vi "MicrofluidicChipControl.vi"() -> ()   [LabVIEW 2023]
uses:
  <vilib>/LabVIEW Interface for Arduino/Type Defs/Board Type.ctl
  <vilib>/LabVIEW Interface for Arduino/Type Defs/Pin Mode.ctl
  <vilib>/LabVIEW Interface for Arduino/LabVIEW Interface for Arduino.lvlib
panel:
  in  "Wait(ms)":dbl=200.0
  in  "Port":refnum<visa-resource-name>="COM3"
  in  "?":string=" BSV4_b"
  in  "?":string=" BSV3_b"
  in  "?":string=" BSV2_b"
  in  "?":string="BSV1_b"
  in  "?":string=" "
  in  "?":string=" "
  in  "?":string="BCV_r"
  in  "?":string="APV_r"
  in  "?":string="CCV"
  in  "?":string="MV"
  in  "?":string="NV"
  in  "?":string="BCV"
  in  "?":string="BV"
  in  "?":string="CRV"
  in  "?":string="SV"
  in  "?":string="SPV"
  in  "?":string="BSV8"
  in  "?":string="BSV7"
  in  "?":string="BSV6"
  in  "?":string="BSV5"
  in  "?":string="BSV4"
  in  "?":string="BSV3"
  in  "?":string="BSV2"
  in  "?":string="BSV1"
  in  "?":string=" COV"
  in  "?":string=" "
  in  "?":string="CCV"
  in  "?":string="CSV4"
  in  "?":string="CSV3"
  in  "?":string="CSV2"
  in  "?":string="CSV1"
  in  "?":string="APV_l"
  in  "D8":bool
  in  "D7":bool
  in  "D6":bool
  in  "D5":bool
  in  "D4":bool
  in  "D3":bool
  in  "D2":bool
  in  "D1":bool
  in  "C8":bool
  in  "C7":bool
  in  "C6":bool
  in  "C5":bool
  in  "C4":bool
  in  "C3":bool
  in  "C2":bool
  in  "C1":bool
  in  "B8":bool
  in  "B7":bool
  in  "B6":bool
  in  "B5":bool
  in  "B4":bool
  in  "B3":bool
  in  "B2":bool
  in  "B1":bool
  in  "A8":bool
  in  "A7":bool
  in  "A6":bool
  in  "A5":bool
  in  "A4":bool
  in  "A3":bool
  in  "A2":bool
  in  "A1":bool
  in  "stop":bool
  in  "Start Mixing":bool
  # "Laboratory of Microtechnologies Applied to Biomedicine"
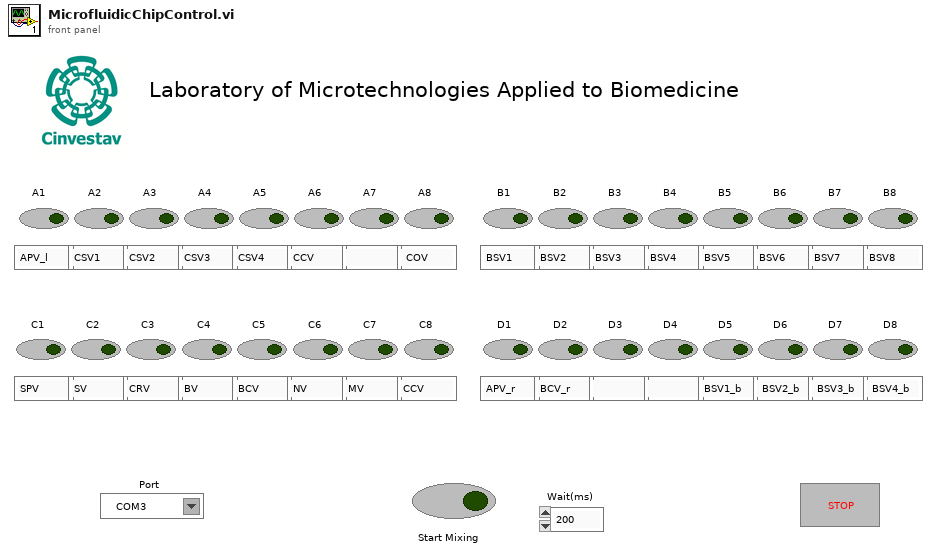
[diagram p1: front panel]
types:
  T1 = typedef "LabVIEW Interface for Arduino.lvlib/Board Type.ctl" = enum16{"Uno", "Dimuelanove w/Atmega 328", "Mega 2560"}
  T2 = typedef "LabVIEW Interface for Arduino.lvlib/Arduino Resource.ctl" = cluster{"VISA resource":refnum<visa-resource-name>, "Board Type":T1, "Connection Type":enum8{"USB / Serial"}, "Bytes Per Packet (15)":u8}
  T3 = typedef "LabVIEW Interface for Arduino.lvlib/Pin Mode.ctl" = enum8{"Input", "Output"}
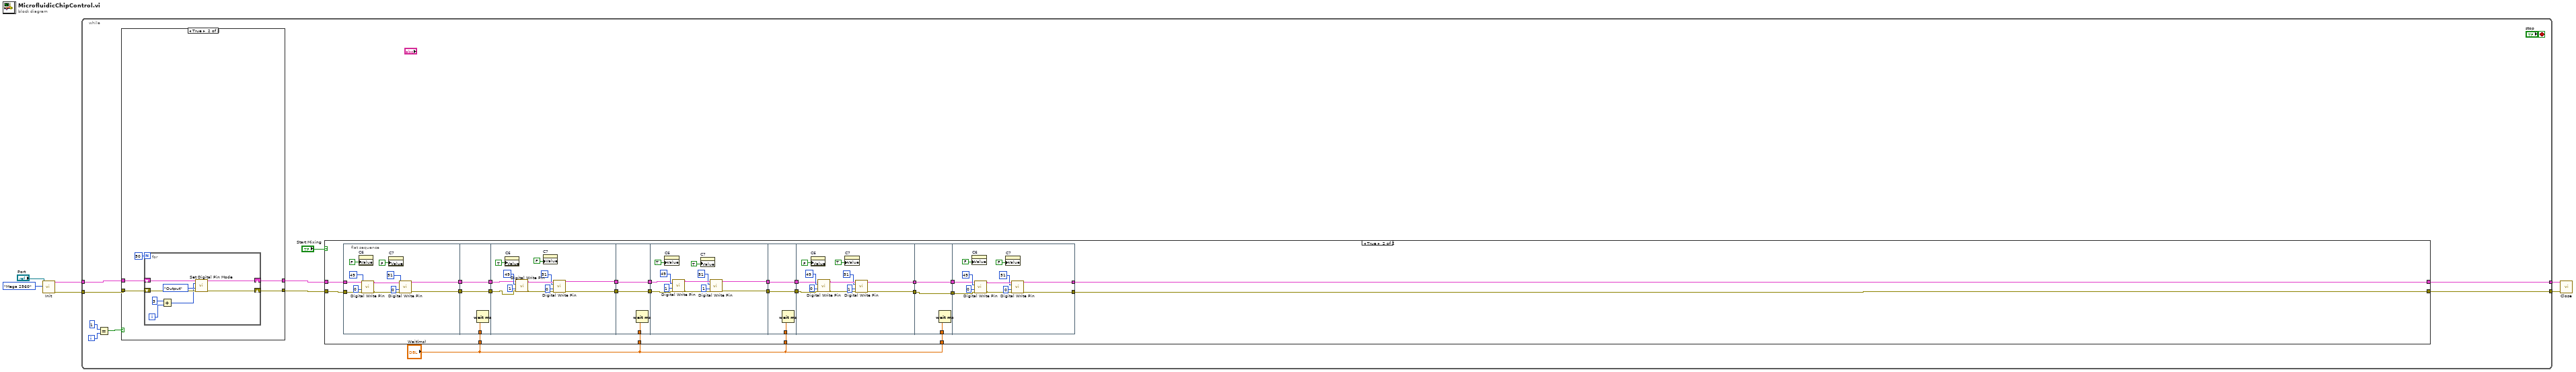
[diagram p0: block diagram]
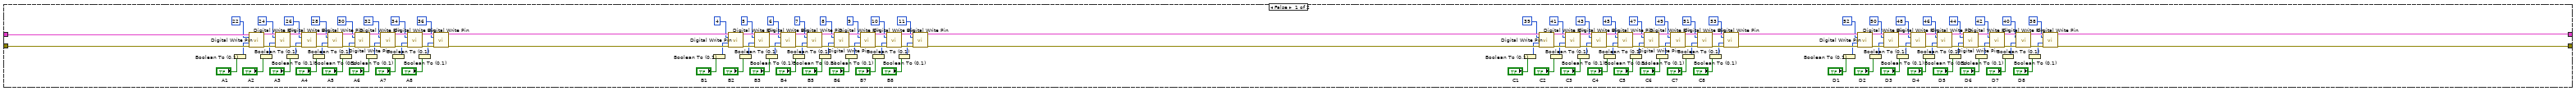
[diagram p2: hidden frame]
diagram:
  n1 = call <vilib>:"Init.vi"("VISA resource"="Port", "Board Type (Uno)"=Board_Type."Mega 2560") -> ("Arduino Resource"=w4:T2, "error out"=w3:errorcluster)  [unwired: 16 in]
  n2 = while {
    tunnel: w4 -> [w15]
    tunnel: w3 -> [w11]
    tunnel: [w10] -> w1
    tunnel: [w9] -> w2
    i -> [w18]
    stop <- "stop" stop-if-true
    n3 = Equal?(x=1, y=w18) -> (x = y?=w16:bool)
    n4 = case shown="True" w16 {
      tunnel: w15 -> [w278 w282]
      tunnel: w11 -> [w277 w281]
      tunnel: [w278 w280] -> w13
      tunnel: [w277 w279] -> w12
      frame False {
      }
      frame True {
        n5 = for {
          N: 50 -> [_]
          shift-right: [w287] -> w280
          shift-left: w282 -> [w290]
          shift-right: [w288] -> w279
          shift-left: w281 -> [w289]
          i -> [w286]
          n6 = Add(x=3, y=w286) -> (x+y=w285:i32)
          n7 = call <vilib>:"Set Digital Pin Mode.vi"("Arduino Resource"=w290, "Digital I/O Pin"=w285, "Pin Mode (Input)"=Pin_Mode."Output", "error in"=w289) -> ("Arduino Resource"=w287:T2, "error out"=w288:errorcluster)  [unwired: 10 in]
        }
      }
    }
    n8 = case shown="True" "Start Mixing" {
      tunnel: w13 -> [w180 w194]
      tunnel: w12 -> [w179 w193]
      tunnel: [w20 w192] -> w9
      tunnel: [w19 w191] -> w10
      tunnel: "Wait(ms)" -> [_ w190]
      tunnel: "Wait(ms)" -> [_ w189]
      tunnel: "Wait(ms)" -> [_ w188]
      tunnel: "Wait(ms)" -> [_ w181]
      frame False {
        n9 = Boolean To (0,1)(Boolean="A1") -> (0, 1=w116:i16)
        n10 = call <vilib>:"Digital Write Pin.vi"("Arduino Resource"=w180, "Digital I/O Pin (0)"=u8 22, "Value (0)"=w116, "error in"=w179) -> ("Arduino Resource"=w178:T2, "error out"=w177:errorcluster)  [unwired: 10 in]
        n11 = Boolean To (0,1)(Boolean="A2") -> (0, 1=w115:i16)
        n12 = call <vilib>:"Digital Write Pin.vi"("Arduino Resource"=w178, "Digital I/O Pin (0)"=u8 24, "Value (0)"=w115, "error in"=w177) -> ("Arduino Resource"=w176:T2, "error out"=w175:errorcluster)  [unwired: 10 in]
        n13 = Boolean To (0,1)(Boolean="A3") -> (0, 1=w114:i16)
        n14 = call <vilib>:"Digital Write Pin.vi"("Arduino Resource"=w176, "Digital I/O Pin (0)"=u8 26, "Value (0)"=w114, "error in"=w175) -> ("Arduino Resource"=w174:T2, "error out"=w173:errorcluster)  [unwired: 10 in]
        n15 = Boolean To (0,1)(Boolean="A4") -> (0, 1=w113:i16)
        n16 = call <vilib>:"Digital Write Pin.vi"("Arduino Resource"=w174, "Digital I/O Pin (0)"=u8 28, "Value (0)"=w113, "error in"=w173) -> ("Arduino Resource"=w172:T2, "error out"=w171:errorcluster)  [unwired: 10 in]
        n17 = Boolean To (0,1)(Boolean="A5") -> (0, 1=w112:i16)
        n18 = call <vilib>:"Digital Write Pin.vi"("Arduino Resource"=w172, "Digital I/O Pin (0)"=u8 30, "Value (0)"=w112, "error in"=w171) -> ("Arduino Resource"=w170:T2, "error out"=w169:errorcluster)  [unwired: 10 in]
        n19 = Boolean To (0,1)(Boolean="A6") -> (0, 1=w111:i16)
        n20 = call <vilib>:"Digital Write Pin.vi"("Arduino Resource"=w170, "Digital I/O Pin (0)"=u8 32, "Value (0)"=w111, "error in"=w169) -> ("Arduino Resource"=w168:T2, "error out"=w167:errorcluster)  [unwired: 10 in]
        n21 = Boolean To (0,1)(Boolean="A7") -> (0, 1=w110:i16)
        n22 = call <vilib>:"Digital Write Pin.vi"("Arduino Resource"=w168, "Digital I/O Pin (0)"=u8 34, "Value (0)"=w110, "error in"=w167) -> ("Arduino Resource"=w166:T2, "error out"=w165:errorcluster)  [unwired: 10 in]
        n23 = Boolean To (0,1)(Boolean="A8") -> (0, 1=w109:i16)
        n24 = call <vilib>:"Digital Write Pin.vi"("Arduino Resource"=w166, "Digital I/O Pin (0)"=u8 36, "Value (0)"=w109, "error in"=w165) -> ("Arduino Resource"=w164:T2, "error out"=w163:errorcluster)  [unwired: 10 in]
        n25 = Boolean To (0,1)(Boolean="B1") -> (0, 1=w108:i16)
        n26 = call <vilib>:"Digital Write Pin.vi"("Arduino Resource"=w164, "Digital I/O Pin (0)"=u8 4, "Value (0)"=w108, "error in"=w163) -> ("Arduino Resource"=w162:T2, "error out"=w161:errorcluster)  [unwired: 10 in]
        n27 = Boolean To (0,1)(Boolean="B2") -> (0, 1=w107:i16)
        n28 = call <vilib>:"Digital Write Pin.vi"("Arduino Resource"=w162, "Digital I/O Pin (0)"=u8 5, "Value (0)"=w107, "error in"=w161) -> ("Arduino Resource"=w160:T2, "error out"=w159:errorcluster)  [unwired: 10 in]
        n29 = Boolean To (0,1)(Boolean="B3") -> (0, 1=w106:i16)
        n30 = call <vilib>:"Digital Write Pin.vi"("Arduino Resource"=w160, "Digital I/O Pin (0)"=u8 6, "Value (0)"=w106, "error in"=w159) -> ("Arduino Resource"=w157:T2, "error out"=w158:errorcluster)  [unwired: 10 in]
        n31 = Boolean To (0,1)(Boolean="B4") -> (0, 1=w105:i16)
        n32 = call <vilib>:"Digital Write Pin.vi"("Arduino Resource"=w157, "Digital I/O Pin (0)"=u8 7, "Value (0)"=w105, "error in"=w158) -> ("Arduino Resource"=w156:T2, "error out"=w155:errorcluster)  [unwired: 10 in]
        n33 = Boolean To (0,1)(Boolean="B5") -> (0, 1=w104:i16)
        n34 = call <vilib>:"Digital Write Pin.vi"("Arduino Resource"=w156, "Digital I/O Pin (0)"=u8 8, "Value (0)"=w104, "error in"=w155) -> ("Arduino Resource"=w154:T2, "error out"=w153:errorcluster)  [unwired: 10 in]
        n35 = Boolean To (0,1)(Boolean="B6") -> (0, 1=w103:i16)
        n36 = call <vilib>:"Digital Write Pin.vi"("Arduino Resource"=w154, "Digital I/O Pin (0)"=u8 9, "Value (0)"=w103, "error in"=w153) -> ("Arduino Resource"=w152:T2, "error out"=w151:errorcluster)  [unwired: 10 in]
        n37 = Boolean To (0,1)(Boolean="B7") -> (0, 1=w102:i16)
        n38 = call <vilib>:"Digital Write Pin.vi"("Arduino Resource"=w152, "Digital I/O Pin (0)"=u8 10, "Value (0)"=w102, "error in"=w151) -> ("Arduino Resource"=w150:T2, "error out"=w149:errorcluster)  [unwired: 10 in]
        n39 = Boolean To (0,1)(Boolean="B8") -> (0, 1=w101:i16)
        n40 = call <vilib>:"Digital Write Pin.vi"("Arduino Resource"=w150, "Digital I/O Pin (0)"=u8 11, "Value (0)"=w101, "error in"=w149) -> ("Arduino Resource"=w118:T2, "error out"=w117:errorcluster)  [unwired: 10 in]
        n41 = Boolean To (0,1)(Boolean="C1") -> (0, 1=w100:i16)
        n42 = call <vilib>:"Digital Write Pin.vi"("Arduino Resource"=w118, "Digital I/O Pin (0)"=u8 39, "Value (0)"=w100, "error in"=w117) -> ("Arduino Resource"=w148:T2, "error out"=w147:errorcluster)  [unwired: 10 in]
        n43 = Boolean To (0,1)(Boolean="C2") -> (0, 1=w99:i16)
        n44 = call <vilib>:"Digital Write Pin.vi"("Arduino Resource"=w148, "Digital I/O Pin (0)"=u8 41, "Value (0)"=w99, "error in"=w147) -> ("Arduino Resource"=w146:T2, "error out"=w145:errorcluster)  [unwired: 10 in]
        n45 = Boolean To (0,1)(Boolean="C3") -> (0, 1=w98:i16)
        n46 = call <vilib>:"Digital Write Pin.vi"("Arduino Resource"=w146, "Digital I/O Pin (0)"=u8 43, "Value (0)"=w98, "error in"=w145) -> ("Arduino Resource"=w144:T2, "error out"=w143:errorcluster)  [unwired: 10 in]
        n47 = Boolean To (0,1)(Boolean="C4") -> (0, 1=w97:i16)
        n48 = call <vilib>:"Digital Write Pin.vi"("Arduino Resource"=w144, "Digital I/O Pin (0)"=u8 45, "Value (0)"=w97, "error in"=w143) -> ("Arduino Resource"=w142:T2, "error out"=w141:errorcluster)  [unwired: 10 in]
        n49 = Boolean To (0,1)(Boolean="C5") -> (0, 1=w96:i16)
        n50 = call <vilib>:"Digital Write Pin.vi"("Arduino Resource"=w142, "Digital I/O Pin (0)"=u8 47, "Value (0)"=w96, "error in"=w141) -> ("Arduino Resource"=w140:T2, "error out"=w139:errorcluster)  [unwired: 10 in]
        n51 = Boolean To (0,1)(Boolean="C6") -> (0, 1=w95:i16)
        n52 = call <vilib>:"Digital Write Pin.vi"("Arduino Resource"=w140, "Digital I/O Pin (0)"=u8 49, "Value (0)"=w95, "error in"=w139) -> ("Arduino Resource"=w138:T2, "error out"=w137:errorcluster)  [unwired: 10 in]
        n53 = Boolean To (0,1)(Boolean="C7") -> (0, 1=w94:i16)
        n54 = call <vilib>:"Digital Write Pin.vi"("Arduino Resource"=w138, "Digital I/O Pin (0)"=u8 51, "Value (0)"=w94, "error in"=w137) -> ("Arduino Resource"=w136:T2, "error out"=w135:errorcluster)  [unwired: 10 in]
        n55 = Boolean To (0,1)(Boolean="C8") -> (0, 1=w93:i16)
        n56 = call <vilib>:"Digital Write Pin.vi"("Arduino Resource"=w136, "Digital I/O Pin (0)"=u8 53, "Value (0)"=w93, "error in"=w135) -> ("Arduino Resource"=w134:T2, "error out"=w133:errorcluster)  [unwired: 10 in]
        n57 = Boolean To (0,1)(Boolean="D1") -> (0, 1=w92:i16)
        n58 = call <vilib>:"Digital Write Pin.vi"("Arduino Resource"=w134, "Digital I/O Pin (0)"=u8 52, "Value (0)"=w92, "error in"=w133) -> ("Arduino Resource"=w132:T2, "error out"=w131:errorcluster)  [unwired: 10 in]
        n59 = Boolean To (0,1)(Boolean="D2") -> (0, 1=w91:i16)
        n60 = call <vilib>:"Digital Write Pin.vi"("Arduino Resource"=w132, "Digital I/O Pin (0)"=u8 50, "Value (0)"=w91, "error in"=w131) -> ("Arduino Resource"=w130:T2, "error out"=w129:errorcluster)  [unwired: 10 in]
        n61 = Boolean To (0,1)(Boolean="D3") -> (0, 1=w90:i16)
        n62 = call <vilib>:"Digital Write Pin.vi"("Arduino Resource"=w130, "Digital I/O Pin (0)"=u8 48, "Value (0)"=w90, "error in"=w129) -> ("Arduino Resource"=w127:T2, "error out"=w128:errorcluster)  [unwired: 10 in]
        n63 = Boolean To (0,1)(Boolean="D4") -> (0, 1=w89:i16)
        n64 = call <vilib>:"Digital Write Pin.vi"("Arduino Resource"=w127, "Digital I/O Pin (0)"=u8 46, "Value (0)"=w89, "error in"=w128) -> ("Arduino Resource"=w126:T2, "error out"=w125:errorcluster)  [unwired: 10 in]
        n65 = Boolean To (0,1)(Boolean="D5") -> (0, 1=w88:i16)
        n66 = call <vilib>:"Digital Write Pin.vi"("Arduino Resource"=w126, "Digital I/O Pin (0)"=u8 44, "Value (0)"=w88, "error in"=w125) -> ("Arduino Resource"=w124:T2, "error out"=w123:errorcluster)  [unwired: 10 in]
        n67 = Boolean To (0,1)(Boolean="D6") -> (0, 1=w87:i16)
        n68 = call <vilib>:"Digital Write Pin.vi"("Arduino Resource"=w124, "Digital I/O Pin (0)"=u8 42, "Value (0)"=w87, "error in"=w123) -> ("Arduino Resource"=w122:T2, "error out"=w121:errorcluster)  [unwired: 10 in]
        n69 = Boolean To (0,1)(Boolean="D7") -> (0, 1=w86:i16)
        n70 = call <vilib>:"Digital Write Pin.vi"("Arduino Resource"=w122, "Digital I/O Pin (0)"=u8 40, "Value (0)"=w86, "error in"=w121) -> ("Arduino Resource"=w120:T2, "error out"=w119:errorcluster)  [unwired: 10 in]
        n71 = Boolean To (0,1)(Boolean="D8") -> (0, 1=w85:i16)
        n72 = call <vilib>:"Digital Write Pin.vi"("Arduino Resource"=w120, "Digital I/O Pin (0)"=u8 38, "Value (0)"=w85, "error in"=w119) -> ("Arduino Resource"=w20:T2, "error out"=w19:errorcluster)  [unwired: 10 in]
      }
      frame True {
        n73 = flat-sequence {
          tunnel: w194 -> [w215]
          tunnel: w193 -> [w214]
          tunnel: [w206] -> w186
          tunnel: [w205] -> w185
          tunnel: [w219] -> w204
          tunnel: [w218] -> w203
          tunnel: w190 -> [w217]
          tunnel: w186 -> [w219]
          tunnel: w185 -> [w218]
          tunnel: w204 -> [w225]
          tunnel: w203 -> [w224]
          tunnel: [w221] -> w201
          tunnel: [w220] -> w199
          tunnel: [w234] -> w202
          tunnel: w201 -> [w234]
          tunnel: [w233] -> w200
          tunnel: w199 -> [w233]
          tunnel: w189 -> [w232]
          tunnel: w202 -> [w239]
          tunnel: w200 -> [w240]
          tunnel: [w236] -> w197
          tunnel: [w235] -> w195
          tunnel: [w249] -> w198
          tunnel: w197 -> [w249]
          tunnel: [w248] -> w196
          tunnel: w195 -> [w248]
          tunnel: w188 -> [w247]
          tunnel: w198 -> [w255]
          tunnel: w196 -> [w254]
          tunnel: [w250] -> w187
          tunnel: [w251] -> w184
          tunnel: w181 -> [w264]
          tunnel: w187 -> [w262]
          tunnel: w184 -> [w263]
          tunnel: [w263] -> w183
          tunnel: [w262] -> w182
          tunnel: w183 -> [w265]
          tunnel: w182 -> [w266]
          tunnel: [w267] -> w191
          tunnel: [w268] -> w192
          frame #0 {
            n74 = property on="C6" class="Bool (strict)"("Value"=FALSE ("C6")) -> ()  [unwired: 2 in, 2 out]
            n75 = call <vilib>:"Digital Write Pin.vi"("Arduino Resource"=w215, "Digital I/O Pin (0)"=u8 49, "Value (0)"=u8 0, "error in"=w214) -> ("Arduino Resource"=w210:T2, "error out"=w209:errorcluster)  [unwired: 10 in]
            n76 = property on="C7" class="Bool (strict)"("Value"=FALSE ("C7")) -> ()  [unwired: 2 in, 2 out]
            n77 = call <vilib>:"Digital Write Pin.vi"("Arduino Resource"=w210, "Digital I/O Pin (0)"=u8 51, "Value (0)"=u8 0, "error in"=w209) -> ("Arduino Resource"=w206:T2, "error out"=w205:errorcluster)  [unwired: 10 in]
          }
          frame #1 {
            n78 = Wait (ms)(milliseconds to wait=w217) -> ()  [unwired: 1 out]
          }
          frame #2 {
            n79 = property on="C6" class="Bool (strict)"("Value"=TRUE ("C6")) -> ()  [unwired: 2 in, 2 out]
            n80 = call <vilib>:"Digital Write Pin.vi"("Arduino Resource"=w225, "Digital I/O Pin (0)"=u8 49, "Value (0)"=u8 1, "error in"=w224) -> ("Arduino Resource"=w230:T2, "error out"=w231:errorcluster)  [unwired: 10 in]
            n81 = property on="C7" class="Bool (strict)"("Value"=FALSE ("C7")) -> ()  [unwired: 2 in, 2 out]
            n82 = call <vilib>:"Digital Write Pin.vi"("Arduino Resource"=w230, "Digital I/O Pin (0)"=u8 51, "Value (0)"=u8 0, "error in"=w231) -> ("Arduino Resource"=w221:T2, "error out"=w220:errorcluster)  [unwired: 10 in]
          }
          frame #3 {
            n83 = Wait (ms)(milliseconds to wait=w232) -> ()  [unwired: 1 out]
          }
          frame #4 {
            n84 = property on="C6" class="Bool (strict)"("Value"=TRUE ("C6")) -> ()  [unwired: 2 in, 2 out]
            n85 = call <vilib>:"Digital Write Pin.vi"("Arduino Resource"=w239, "Digital I/O Pin (0)"=u8 49, "Value (0)"=u8 1, "error in"=w240) -> ("Arduino Resource"=w246:T2, "error out"=w245:errorcluster)  [unwired: 10 in]
            n86 = property on="C7" class="Bool (strict)"("Value"=TRUE ("C7")) -> ()  [unwired: 2 in, 2 out]
            n87 = call <vilib>:"Digital Write Pin.vi"("Arduino Resource"=w246, "Digital I/O Pin (0)"=u8 51, "Value (0)"=u8 1, "error in"=w245) -> ("Arduino Resource"=w236:T2, "error out"=w235:errorcluster)  [unwired: 10 in]
          }
          frame #5 {
            n88 = Wait (ms)(milliseconds to wait=w247) -> ()  [unwired: 1 out]
          }
          frame #6 {
            n89 = property on="C6" class="Bool (strict)"("Value"=FALSE ("C6")) -> ()  [unwired: 2 in, 2 out]
            n90 = call <vilib>:"Digital Write Pin.vi"("Arduino Resource"=w255, "Digital I/O Pin (0)"=u8 49, "Value (0)"=u8 0, "error in"=w254) -> ("Arduino Resource"=w261:T2, "error out"=w260:errorcluster)  [unwired: 10 in]
            n91 = property on="C7" class="Bool (strict)"("Value"=TRUE ("C7")) -> ()  [unwired: 2 in, 2 out]
            n92 = call <vilib>:"Digital Write Pin.vi"("Arduino Resource"=w261, "Digital I/O Pin (0)"=u8 51, "Value (0)"=u8 1, "error in"=w260) -> ("Arduino Resource"=w251:T2, "error out"=w250:errorcluster)  [unwired: 10 in]
          }
          frame #7 {
            n93 = Wait (ms)(milliseconds to wait=w264) -> ()  [unwired: 1 out]
          }
          frame #8 {
            n94 = property on="C6" class="Bool (strict)"("Value"=FALSE ("C6")) -> ()  [unwired: 2 in, 2 out]
            n95 = call <vilib>:"Digital Write Pin.vi"("Arduino Resource"=w265, "Digital I/O Pin (0)"=u8 49, "Value (0)"=u8 0, "error in"=w266) -> ("Arduino Resource"=w275:T2, "error out"=w276:errorcluster)  [unwired: 10 in]
            n96 = property on="C7" class="Bool (strict)"("Value"=FALSE ("C7")) -> ()  [unwired: 2 in, 2 out]
            n97 = call <vilib>:"Digital Write Pin.vi"("Arduino Resource"=w275, "Digital I/O Pin (0)"=u8 51, "Value (0)"=u8 0, "error in"=w276) -> ("Arduino Resource"=w268:T2, "error out"=w267:errorcluster)  [unwired: 10 in]
          }
        }
      }
    }
  }
  n98 = call <vilib>:"Close.vi"("Arduino Resource"=w2, "error in"=w1) -> ()  [unwired: 13 in, 1 out]
